vi "Setup.vi"(11 "Transport in":refnum<class "Transport.lvclass">) -> (0 "Error out":errorcluster, 3 "Transport out":refnum<class "Transport.lvclass">)   [LabVIEW 2025, in "jettl.lvlib" / "Transport.lvlib" / "Transport.lvclass"]
uses:
  Transport.lvclass
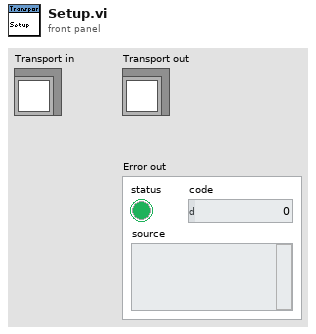
[diagram p1: front panel]
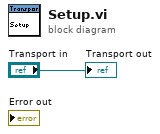
[diagram p0: block diagram]
diagram:
  "Transport out" <- "Transport in"
